vi "1mhzabstimingsource_1000dt.vi"() -> (0 "max jitter (uS)":dbl format="%.2f", 1 "mean time (uS)":dbl format="%.2f", 2 "standard deviation (uS)":dbl format="%.2f", 3 "execution histogram":T1(graph), 4 "Error":errorcluster, 5 "execution times (uS)":dbl[](graph))   [LabVIEW 2013]
uses:
  <vilib>/Platform/TimedLoop/XDataNode/timing_clust.ctl
  <vilib>/Platform/TimedLoop/XDataNode/nitl_modes.ctl
  <vilib>/Platform/TimedLoop/XDataNode/wakeup.ctl
  <vilib>/Platform/TimedLoop/TimeConversion.llb/rt-rel-time-to-microseconds.vi
  <vilib>/Platform/TimedLoop/TimeConversion.llb/rt-timestamp-to-microseconds.vi
  <vilib>/Platform/TimedLoop/TimeConversion.llb/rt-microseconds-to-timestamp.vi
  <vilib>/platform/TimedLoop/XDataNode/XDataNode.xnode
  <vilib>/Platform/TimedLoop/XDataNode/XDNodeRunTimeDep.lvlib
  <vilib>/NI_Real-Time Target Support.lvlib
panel:
  out "Error 2":errorcluster
  out "x-y":dbl
  out "current time":timestamp
  out "act":timestamp
  out "start":timestamp
  out "Numeric":i32=-1
  out "actual":dbl format="%#_32f"
  out "desired":dbl format="%#_32f"
  out "diff":dbl format="%#_32f"
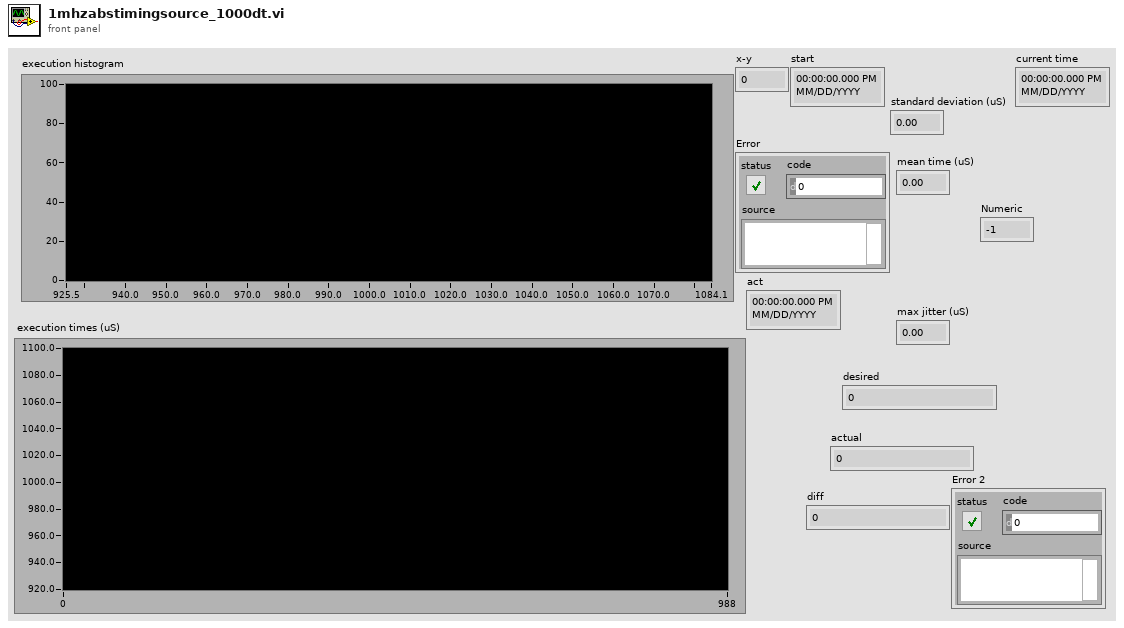
[diagram p1: front panel]
types:
  T1 = cluster{"X Values":dbl[], "Histogram: h(x)":i32[]}
  T2 = typedef "XDNodeRunTimeDep.lvlib/timing_clust.ctl" = cluster{"Expected End [f-1]":u64, "Actual End [f-1]":u64, "Finished Late? [f-1]":bool, "Expected End [i-1]":u64, "Actual End [i-1]":u64, "Finished Late? [i-1]":bool, "Expected Start [i]":u64, "Actual Start [i]":u64, "Expected Start [f]":u64, "Actual Start [f]":u64, "Source Name":string, "Structure Name":string, "Period":i64, "Deadline":i64, "Offset":i64, "Start":i64, "Priority":i32, "Timeout":i32, "Mode":T3, "Wakeup Reason":T4, "Error":errorcluster, "Source Type":string, "Secondary Source Type":string, "Global End Time":u64, "Global Start Time":u64, "Frame Duration":u64, "Iteration Duration":u64, "Assigned CPU":i32, "I/O Scan Engine Mode":u32}
  T3 = typedef "XDNodeRunTimeDep.lvlib/nitl_modes.ctl" = enum32{"No Change", "Process missed periods, maintain original phase", "Discard missed periods, maintain original phase", "Process missed periods, ignore original phase", "Discard missed periods, ignore original phase"}
  T4 = typedef "XDNodeRunTimeDep.lvlib/wakeup.ctl" = enum32{"Normal", "Aborted", "Asynchronous wakeup", "Timing source error", "Timed loop error", "Timeout"}
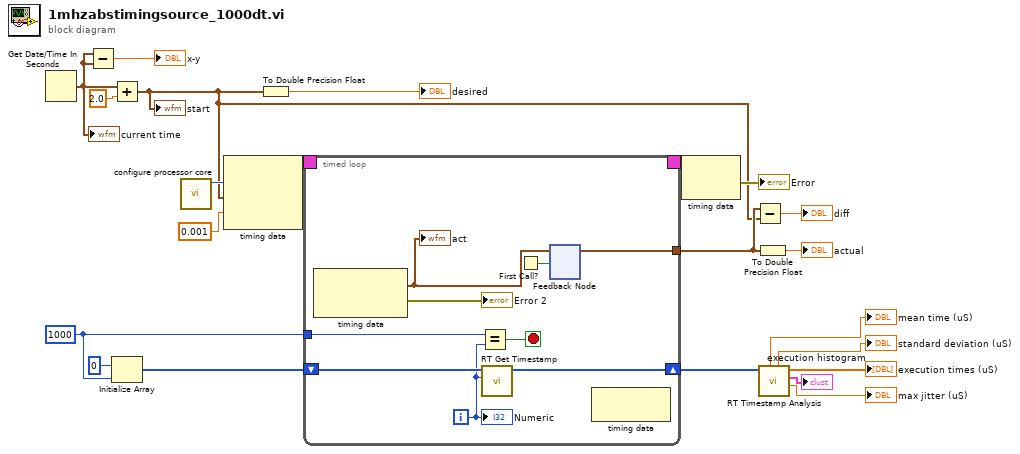
[diagram p0: block diagram]
diagram:
  w20 = 1000 ("x")
  n1 = Get Date/Time In Seconds() -> (seconds since 1Jan1904=w3:timestamp)
  "current time" <- w3
  n2 = Subtract(x=w3, y=w3) -> (x-y=→"x-y":dbl)
  n3 = Add(x=w3, y=2.0) -> (x+y=w1:timestamp)
  "start" <- w1
  n4 = Initialize Array(u64 0, w20) -> (w21:u64[])
  n5 = call "configure processor core.vi"() -> ("Processor"=w10:i32)  [unwired: 11 in]
  n6 = node-c288(w10, w1, 0.001) -> (w13:T2)
  n7 = To Double Precision Float(number=w1) -> (double precision float=→"desired":dbl)
  n8 = timed-loop {
    timing: w13 -> [_]
    timing-out: [_] -> w12
    shift-right: [w28] -> w19
    shift-left: w21 -> [w29]
    tunnel: w20 -> [w31]
    tunnel: [w26] -> w5
    i -> [w27]
    stop <- w30 stop-if-true
    n9 = node-c288() -> (w24:timestamp, →"Error 2":errorcluster)  [unwired: 1 in]
    "act" <- w24
    n10 = Equal?(x=w31, y=w27) -> (x = y?=w30:bool)
    n11 = call <vilib>:"RT Get Timestamp.vi"("iteration"=w27, "timestamp array in"=w29) -> ("timestamp array out"=w28:u64[])  [unwired: 8 in, 1 out]
    n12 = First Call?() -> (First Call?: T/F=w25:bool)
    n13 = feedback-in #1(w24, w25) -> ()
    n14 = feedback #1() -> (w26:timestamp)  [unwired: 1 in]
    n15 = node-c288() -> ()  [unwired: 1 in, 1 out]
    "Numeric" <- w27
  }
  n16 = node-c288(w12) -> (→"Error":errorcluster)
  n17 = Subtract(x=w5, y=w1) -> (x-y=→"diff":dbl)
  n18 = To Double Precision Float(number=w5) -> (double precision float=→"actual":dbl)
  n19 = call <vilib>:"RT Timestamp Analysis.vi"("timestamp array"=w19) -> ("max jitter (uS)"=→"max jitter (uS)":dbl, "execution histogram"=→"execution histogram":T1, "execution times (uS)"=→"execution times (uS)":dbl[], "standard deviation (uS)"=→"standard deviation (uS)":dbl, "mean time (uS)"=→"mean time (uS)":dbl)  [unwired: 5 in, 1 out]
